vi "Calculate Particle Scores.vi"(7 "Pixel Value":i32=1, 8 "Limit Tests?":bool=TRUE, 9 "Aspect Fudge Factor":dbl=1.0, 10 "Sorted Data":dbl[][](array[numeric]), 11 "Image in":T2) -> (3 "Scores":T1(array[cluster]))   [LabVIEW 2015]
doc: "Calculate scores based on the particle measurements. Calculated scores are for aspect ratio, area to convex hull area, masking, and moment of inertia. These scores range between 0 and 100 and can be used to categorize particles as targets and non-targets. The fudge factor compensates for camera modes that do not give square pixels."
uses:
  <vilib>/vision/Image Controls.llb/IMAQ Image.ctl
  <vilib>/vision/NI_Vision_Development_Module.lvlib
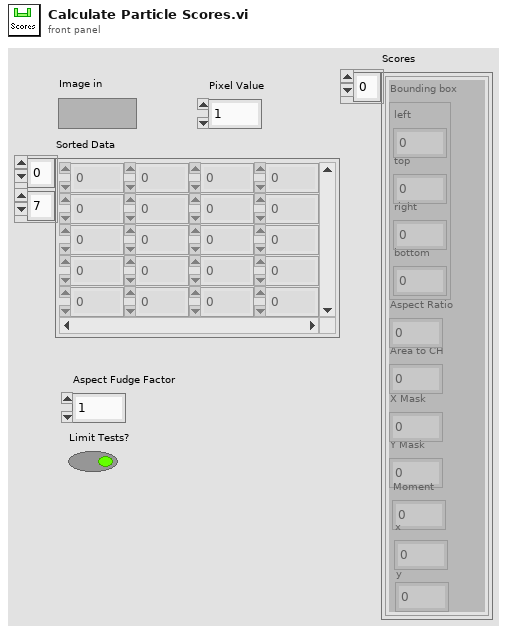
[diagram p1: front panel]
types:
  T1 = cluster{"Bounding box":cluster{"left":dbl, "top":dbl, "right":dbl, "bottom":dbl}, "Aspect Ratio":dbl, "Area to CH":dbl, "X Mask":dbl, "Y Mask":dbl, "Moment":dbl, "x":dbl, "y":dbl}[]
  T2 = typedef "IMAQ Image.ctl" = refnum<image>
  T3 = cluster{"[0]":dbl, "[1]":dbl, "[2]":dbl, "[3]":dbl}
  T4 = cluster{cluster{"[0]":dbl, "[1]":dbl, "[2]":dbl, "[3]":dbl}, "Aspect Ratio Score":dbl, "Score":dbl, "X Score":dbl, "Y Score":dbl, "Score":dbl, "Numeric":dbl, "Numeric":dbl}
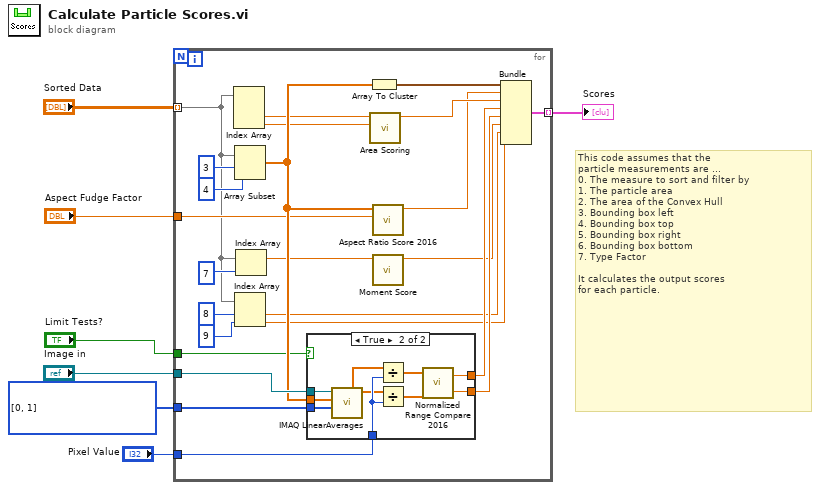
[diagram p0: block diagram]
diagram:
  w5 = i32[] [0, 1] items=["X Axis Averages", "Y Axis Averages", "X + Y Axis Averages", "X - Y Axis Averages"] ("Averages")
  # "This code assumes that the\nparticle measurements are ...\n0. The measure to sort and filter by\n1. The particle area\n2. The area of the Convex Hull\n3. Bounding box left\n4. Bounding box top\n5. Bounding box right\n6. Bounding box bottom\n7. Type Factor\n\nIt calculates the output scores\nfor each particle."
  n1 = for {
    tunnel: "Image in" -> [w27]
    tunnel: "Sorted Data" -> [w10] mode=indexing
    tunnel: [w29] -> w6 mode=indexing
    tunnel: w5 -> [w22]
    tunnel: "Pixel Value" -> [w20]
    tunnel: "Aspect Fudge Factor" -> [w17]
    tunnel: "Limit Tests?" -> [w16]
    n2 = Index Array(array=w10) -> (element #2=w19:dbl, element #3=w18:dbl)  [unwired: 3 in, 1 out]
    n3 = Array Subset(array=w10, index=3, length=4) -> (w21:dbl[])
    n4 = Index Array(array=w10, index #1=8 ("index"), index #2=9 ("index")) -> (element #1=w9:dbl, element #2=w8:dbl)
    n5 = Index Array(array=w10, index=7 ("length")) -> (element=w14:dbl)
    n6 = case shown="True" w16 {
      tunnel: w27 -> [_ w41]
      tunnel: [_ w40] -> w24
      tunnel: [_ w39] -> w23
      tunnel: w22 -> [_ w38]
      tunnel: w21 -> [_ w37]
      tunnel: w20 -> [_ w36]
      frame False {
      }
      frame True {
        n7 = call "IMAQ LinearAverages"("Averages"=w38, "Optional Rectangle"=w37, "Image Src"=w41) -> ("Y Axis Averages"=w34:sgl[], "X Axis Averages"=w35:sgl[])  [unwired: 4 in, 3 out]
        n8 = Divide(x=w35, y=w36) -> (x/y=w33:sgl[])
        n9 = Divide(x=w34, y=w36) -> (x/y=w32:sgl[])
        n10 = call "Normalized Range Compare 2016.vi"("Y Averages"=w32, "X Averages"=w33) -> ("Y Score"=w39:dbl, "X Score"=w40:dbl)
      }
    }
    n11 = Array To Cluster(array=w21) -> (cluster=w26:T3)
    n12 = call "Area Scoring.vi"("Convex Hull Area"=w18, "Area"=w19) -> ("Score"=w28:dbl)  [unwired: 9 in]
    n13 = call "Aspect Ratio Score 2016.vi"("Aspect Fudge Factor"=w17, "Rectangle Array ltrb"=w21) -> ("Aspect Ratio Score"=w25:dbl)  [unwired: 9 in]
    n14 = call "Moment Score.vi"("Moment Factor"=w14) -> ("Score"=w13:dbl)  [unwired: 10 in]
    n15 = Bundle(w26, "Aspect Ratio Score"=w25, "Score"=w28, "X Score"=w24, "Y Score"=w23, "Score"=w13, "Numeric"=w9, "Numeric"=w8) -> (w29:T4)  [unwired: 1 in]
  }
  "Scores" <- w6
